vi "Qpori.vi"(2 "Dt":dbl, 3 "Numeric":i32, 4 "Dn":dbl) -> (0 "pori":dbl, 1 "Q":dbl)   [LabVIEW 2018]
panel:
  out "output variable 2":dbl
  out "output variable":dbl
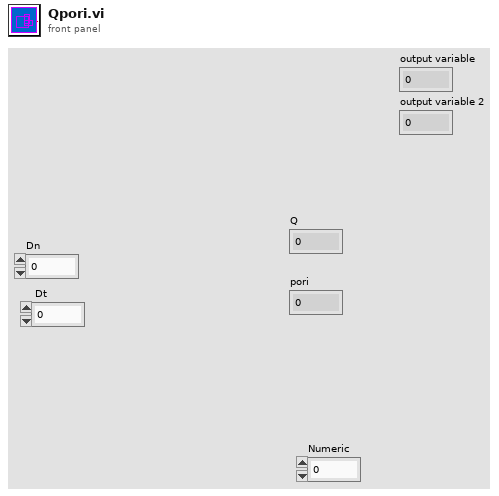
[diagram p1: front panel]
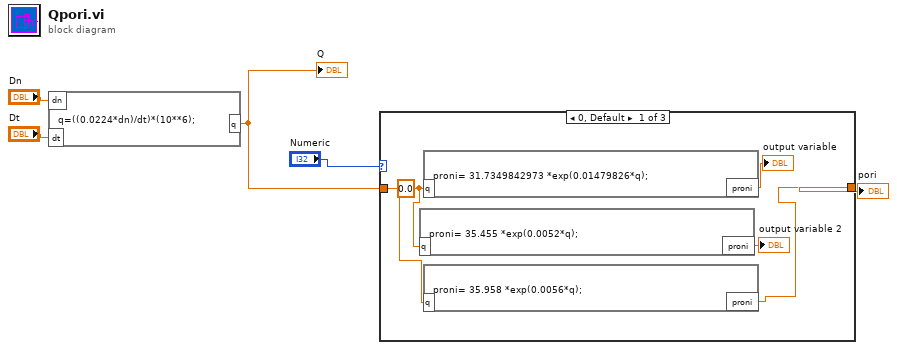
[diagram p0: block diagram]
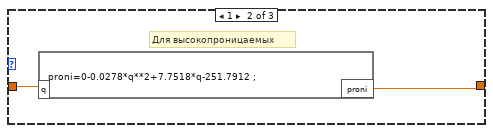
[diagram p2: hidden frame]
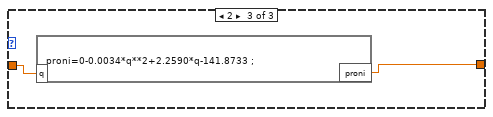
[diagram p3: hidden frame]
diagram:
  n1 = formula code="q=((0.0224*dn)/dt)*(10**6);"("dn"="Dn", "dt"="Dt") -> ("q"=w2:dbl)
  "Q" <- w2
  n2 = case shown="0, Default" "Numeric" {
    tunnel: [w6 w12 w13] -> w5
    tunnel: w2 -> [w10 w11 w14]
    frame 0, Default {
      w9 = 0.0 ("input variable")
      n3 = formula code="proni= 35.455 *exp(0.0052*q);"("q"=w9) -> ("proni"=→"output variable 2":dbl)
      n4 = formula code="proni= 31.7349842973 *exp(0.01479826*q);"("q"=w9) -> ("proni"=→"output variable":dbl)
      n5 = formula code="proni= 35.958 *exp(0.0056*q);"("q"=w10) -> ("proni"=w6:dbl)
    }
    frame 1 {
      # "Для высокопроницаемых"
      n6 = formula code="proni=0-0.0278*q**2+7.7518*q-251.7912 ;"("q"=w11) -> ("proni"=w12:dbl)
    }
    frame 2 {
      n7 = formula code="proni=0-0.0034*q**2+2.2590*q-141.8733 ;"("q"=w14) -> ("proni"=w13:dbl)
    }
  }
  "pori" <- w5
